vi "GetVIFolderPath.vi"(8 "error in (no error)":errorcluster, 11 "VI Reference in":refnum<vi>) -> (0 "error out":errorcluster, 3 "VI Folder Path out":path)   [LabVIEW 2027, in "VeriStandTestUtilities.lvlib"]
uses:
  VeriStandTestUtilities.lvlib
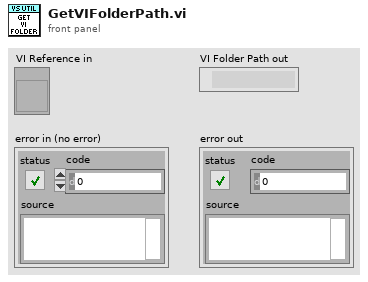
[diagram p1: front panel]
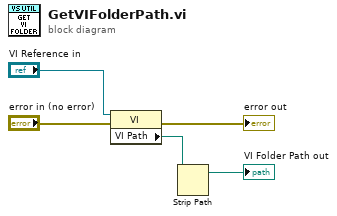
[diagram p0: block diagram]
diagram:
  n1 = property class="VI"(reference="VI Reference in", error in="error in (no error)") -> (error out=→"error out":errorcluster, "VI Path"=w5:path)  [unwired: 1 out]
  n2 = Strip Path(path=w5) -> (stripped path=→"VI Folder Path out":path)  [unwired: 1 out]
